vi "采配水启动命令.vi"(8 "error in (no error)":errorcluster, 11 "启动/停止命令":T1(ring)) -> (0 "error out":errorcluster)   [LabVIEW 2016, in "质控单元V2.lvlib"]
uses:
  <vilib>/Plasmionique/MB Master/MB Master.lvlib
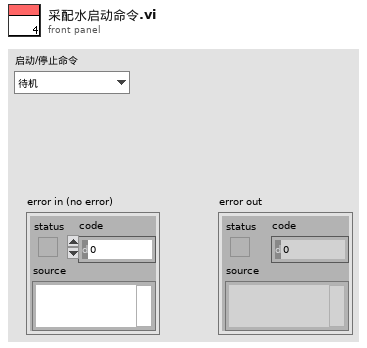
[diagram p1: front panel]
types:
  T1 = enum16{"待机", "水样测试（全流程）", "停止", "加标回收", "水样测试（简易流程）"}
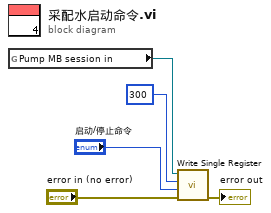
[diagram p0: block diagram]
diagram:
  n1 = global read "系统交互.vi" "Pump MB session in"() -> (w3:refnum<class "MB_Master.lvclass">)
  n2 = call <vilib>:"Write Single Register.vi"("error in (no error)"="error in (no error)", "value"="启动/停止命令", "address"=u16 300 ("starting address"), "MB session in"=w3) -> ("error out"=→"error out":errorcluster)  [unwired: 6 in, 1 out]
